vi "Read AVI File.vi"() -> ()   [LabVIEW 2014]
doc: "This example shows how to open, read, and display an AVI file in NI Vision. The VI reads the frames per second property and plays the images back at the rate specified by the AVI file."
panel:
  out "Progress Bar":i32(slide) max=135 scale=1.0..135.0
  in  "Stop":bool
  out "Image":T1(plugin-control)
  # "Overview: Demonstrate the use of the AVI functions to read an AVI movie file.\nRequirements: Vision Development Software.\nInstructions: Run the VI."
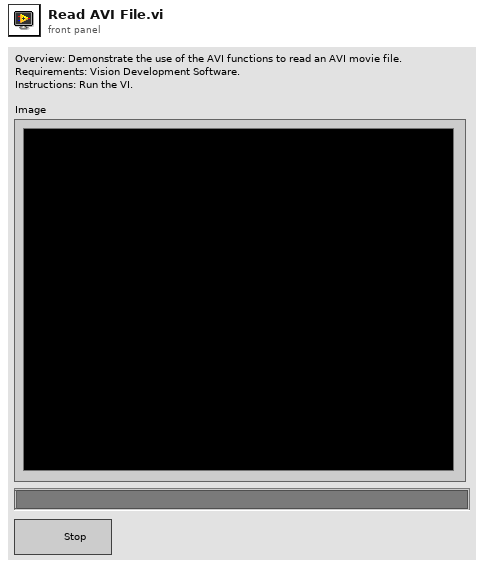
[diagram p1: front panel]
types:
  T1 = typedef "IMAQ Image.ctl" = refnum<image>
  T2 = typedef "IMAQ AVI2 Refnum.ctl" = refnum<k20>
  T3 = typedef "Image Type" = u32
  T4 = cluster{"Width":u32, "Height":u32, "Frames Per Second":u32, "Codec":string, "Has Data":bool}
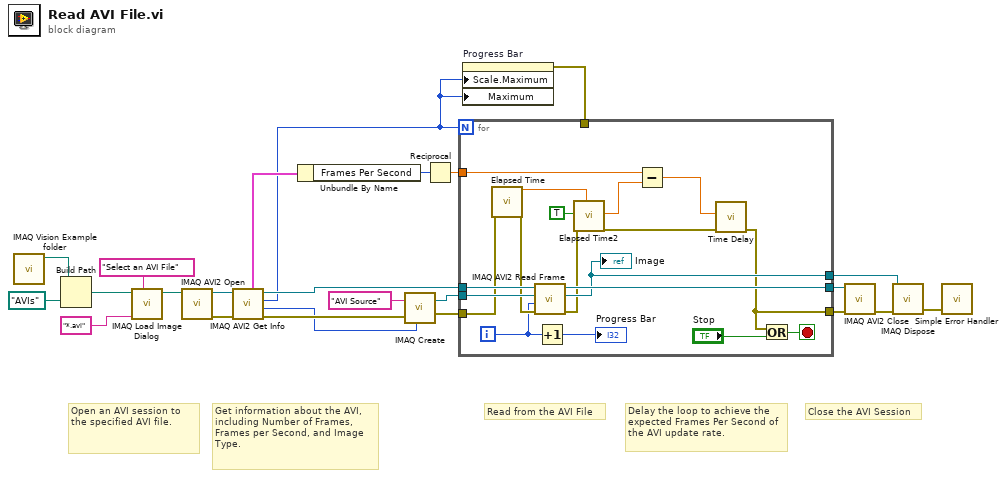
[diagram p0: block diagram]
diagram:
  # "Close the AVI Session"
  # "Read from the AVI File"
  # "Get information about the AVI, including Number of Frames, Frames per Second, and Image Type."
  # "Open an AVI session to the specified AVI file."
  # "Delay the loop to achieve the expected Frames Per Second of the AVI update rate."
  n1 = call "IMAQ Vision Example folder.vi"() -> ("Example Image Path"=w8:path)  [unwired: 11 in]
  n2 = Build Path(base path=w8, name or relative path=path "AVIs") -> (appended path=w5:path)
  n3 = call "IMAQ Load Image Dialog"("Prompt"="Select an AVI File" ("prompt"), "Pattern"="*.avi", "Start Path"=w5) -> ("Path"=w4:path)  [unwired: 6 in, 2 out]
  n4 = call "IMAQ AVI2 Open"("AVI File Path"=w4) -> ("error out"=w21:errorcluster, "AVI Refnum"=w20:T2)  [unwired: 2 in, 7 out]
  n5 = call "IMAQ AVI2 Get Info"("error in (no error)"=w21, "AVI Refnum"=w20) -> ("error out"=w17:errorcluster, "Image Type"=w11:T3, "Number of Frames"=w2:u32, "AVI Refnum (duplicate)"=w14:T2, "Frame Data"=w22:T4)  [unwired: 5 out]
  n6 = Unbundle By Name(w22) -> ("Frames Per Second"=w10:u32)
  n7 = call "IMAQ Create"("Image Name"="AVI Source", "Image Type"=w11, "error in (no error)"=w17) -> ("New Image"=w15:T1, "error out"=w16:errorcluster)  [unwired: 1 in, 1 out]
  n8 = Reciprocal(x=w10) -> (1/x=w9:dbl)
  n9 = property on="Progress Bar" class="Slide (strict)"("Scale.Maximum"=w2, "Maximum"=w2) -> (error out=w1:errorcluster)  [unwired: 2 in, 1 out]
  n10 = for {
    N: w2 -> [_]
    tunnel: w15 -> [w41]
    tunnel: [w40] -> w18
    tunnel: [w29] -> w19
    tunnel: w16 -> [w39]
    tunnel: w14 -> [w42]
    tunnel: [w35] -> w12
    tunnel: w9 -> [w37]
    tunnel: w1 -> [_]
    i -> [w26]
    stop <- w27 stop-if-true
    n11 = call "Elapsed Time"("error in (no error)"=w39) -> ("Present (s)"=w34:dbl, "error out"=w38:errorcluster)  [unwired: 11 in, 6 out]
    n12 = call "IMAQ AVI2 Read Frame"("error in (no error)"=w38, "Frame Number"=w26, "Image"=w41, "AVI Refnum"=w42) -> ("error out"=w32:errorcluster, "Image Out"=w35:T1, "AVI Refnum (duplicate)"=w40:T2)  [unwired: 5 out]
    "Image" <- w35
    n13 = Increment(x=w26) -> (x+1=→"Progress Bar":i32)
    n14 = call "Elapsed Time2"("Reset"=TRUE, "error in (no error)"=w32, "Set Start Time (s)"=w34) -> ("Elapsed Time (s)"=w31:dbl, "error out"=w30:errorcluster)  [unwired: 9 in, 6 out]
    n15 = Subtract(x=w37, y=w31) -> (x-y=w36:dbl)
    n16 = call "Time Delay"("error in (no error)"=w30, "Delay Time (s)"=w36) -> ("error out"=w29:errorcluster)  [unwired: 9 in]
    n17 = Or(x=w29, y="Stop") -> (x .or. y?=w27:bool)
  }
  n18 = call "IMAQ AVI2 Close"("error in (no error)"=w19, "AVI Refnum"=w18) -> ("error out"=w13:errorcluster)  [unwired: 9 out]
  n19 = call "IMAQ Dispose"("Image"=w12, "error in (no error)"=w13) -> ("error out"=w23:errorcluster)  [unwired: 1 in, 3 out]
  n20 = call <vilib>:"Simple Error Handler.vi"("error in (no error)"=w23) -> ()  [unwired: 1 in, 8 out]
